vi "input.vi"(8 "error in":errorcluster, 10 "data table in":T1, 11 "UI Reference runtime in":refnum<class "UI Reference runtime.lvclass">) -> (0 "error out":errorcluster, 2 "data table out":T1, 3 "UI Reference runtime out":refnum<class "UI Reference runtime.lvclass">)   [LabVIEW 2013, in "UI Reference runtime.lvclass"]
doc: "Provides an interface for reading data from a module at runtime. While this interface performs no operations, a child should provide an override which may read from any open sessions, references, or interfaces."
uses:
  UI Reference runtime.lvclass
  <vilib>/NI/Tag Bus/table/data table.ctl
  UI Reference runtime.lvclass/UI Reference runtime.ctl
  <vilib>/NI/Tag Bus/table/data polymorphs/write many/write Doubles.vi
  <vilib>/NI/Tag Bus/table/data polymorphs/write many/write Singles.vi
  <vilib>/NI/Tag Bus/table/data polymorphs/write many/write I64s.vi
  <vilib>/NI/Tag Bus/table/data polymorphs/write many/write I32s.vi
  <vilib>/NI/Tag Bus/table/data polymorphs/write many/write I16s.vi
  <vilib>/NI/Tag Bus/table/data polymorphs/write many/write I8s.vi
  <vilib>/NI/Tag Bus/table/data polymorphs/write many/write U64s.vi
  <vilib>/NI/Tag Bus/table/data polymorphs/write many/write U32s.vi
  <vilib>/NI/Tag Bus/table/data polymorphs/write many/write U16s.vi
  <vilib>/NI/Tag Bus/table/data polymorphs/write many/write U8s.vi
  <vilib>/NI/Tag Bus/table/data polymorphs/write many/write Booleans.vi
  <vilib>/NI/Tag Bus/table/data polymorphs/write many/write Strings.vi
  <vilib>/NI/Tag Bus/table/data polymorphs/write one/write Array of Double.vi
  <vilib>/NI/Tag Bus/table/data polymorphs/write one/write Array of Single.vi
  <vilib>/NI/Tag Bus/table/data polymorphs/write one/write Array of I64.vi
  <vilib>/NI/Tag Bus/table/data polymorphs/write one/write Array of I32.vi
  <vilib>/NI/Tag Bus/table/data polymorphs/write one/write Array of I16.vi
  <vilib>/NI/Tag Bus/table/data polymorphs/write one/write Array of I8.vi
  <vilib>/NI/Tag Bus/table/data polymorphs/write one/write Array of U64.vi
  <vilib>/NI/Tag Bus/table/data polymorphs/write one/write Array of U32.vi
  <vilib>/NI/Tag Bus/table/data polymorphs/write one/write Array of U16.vi
  <vilib>/NI/Tag Bus/table/data polymorphs/write one/write Array of U8.vi
  <vilib>/NI/Tag Bus/table/data polymorphs/write one/write Array of Boolean.vi
  <vilib>/NI/Tag Bus/table/data polymorphs/write one/write Array of String.vi
  <vilib>/NI/Tag Bus/table/data table.lvlib
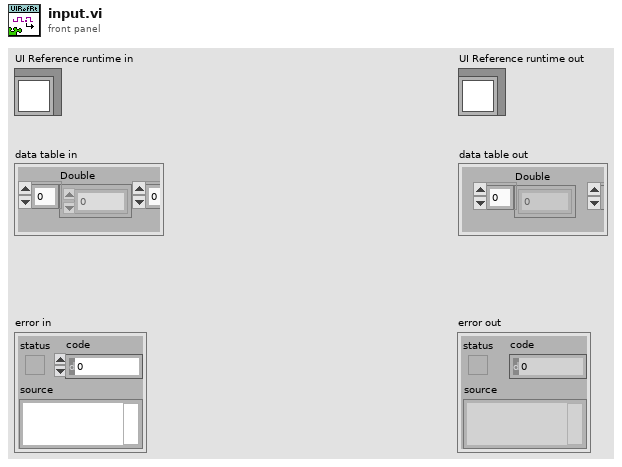
[diagram p1: front panel]
types:
  T1 = typedef "tag bus.lvlib/data table.lvlib/data table.ctl" = cluster{"Double":dbl[], "Single":sgl[], "I64":i64[], "I32":i32[], "I16":i16[], "I8":i8[], "U64":u64[], "U32":u32[], "U16":u16[], "U8":u8[], "Boolean":bool[], "String":string[], "Array of Double":cluster{"DBL Array":dbl[]}[], "Array of Single":cluster{"SGL Array":sgl[]}[], "Array of I64":cluster{"I64 Array":i64[]}[], "Array of I32":cluster{"I32 Array":i32[]}[], "Array of I16":cluster{"I16 Array":i16[]}[], "Array of I8":cluster{"I8 Array":i8[]}[], "Array of U64":cluster{"U64 Array":u64[]}[], "Array of U32":cluster{"U32 Array":u32[]}[], "Array of U16":cluster{"U16 Array":u16[]}[], "Array of U8":cluster{"U8 Array":u8[]}[], "Array of Boolean":cluster{"Boolean Array":bool[]}[], "Array of String":cluster{"String Array":string[]}[]}
  T2 = typedef "UI Reference runtime.lvclass/control index set.ctl" = cluster{"data type":T3, "control indexes":i32[], "data indexes":i32[]}
  T3 = typedef "tag bus.lvlib/tag descriptor.lvclass/Data Type.ctl" = enum16{"Double", "Single", "I64", "I32", "I16", "I8", "U64", "U32", "U16", "U8", "Boolean", "String", "Array of Double", "Array of Single", "Array of I64", "Array of I32", "Array of I16", "Array of I8", "Array of U64", "Array of U32", "Array of U16", "Array of U8", "Array of Boolean", "Array of String"}
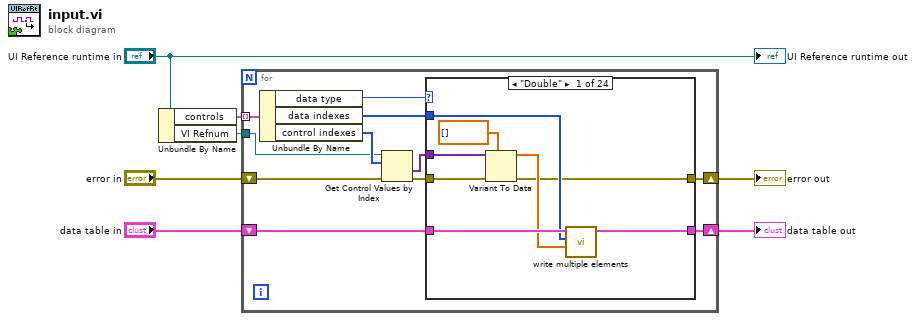
[diagram p0: block diagram]
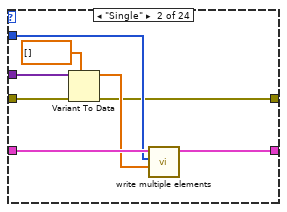
[diagram p2: hidden frame]
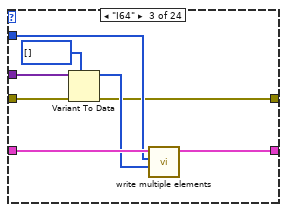
[diagram p3: hidden frame]
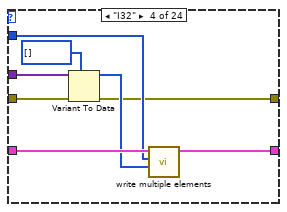
[diagram p4: hidden frame]
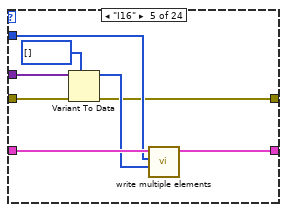
[diagram p5: hidden frame]
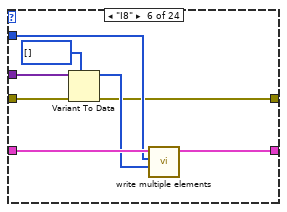
[diagram p6: hidden frame]
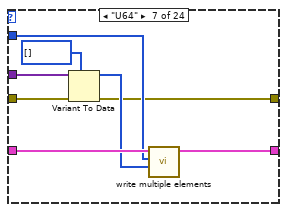
[diagram p7: hidden frame]
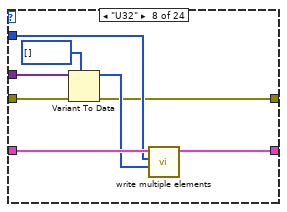
[diagram p8: hidden frame]
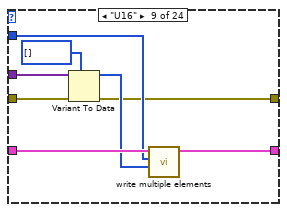
[diagram p9: hidden frame]
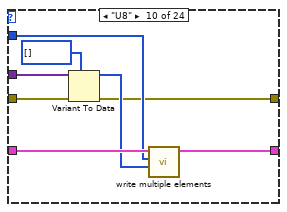
[diagram p10: hidden frame]
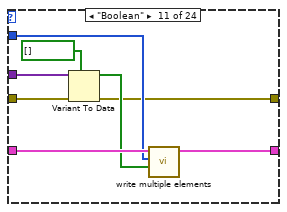
[diagram p11: hidden frame]
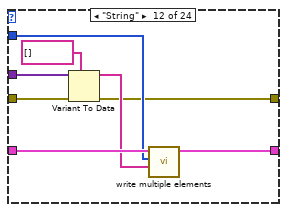
[diagram p12: hidden frame]
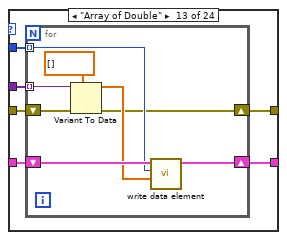
[diagram p13: hidden frame]
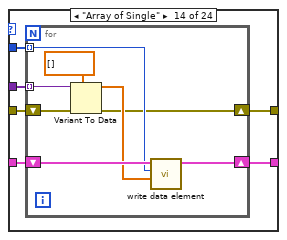
[diagram p14: hidden frame]
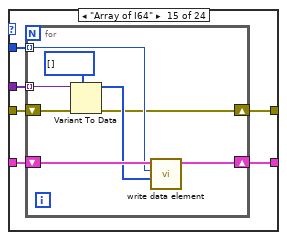
[diagram p15: hidden frame]
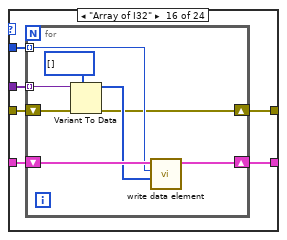
[diagram p16: hidden frame]
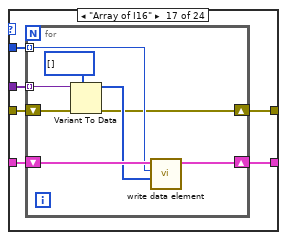
[diagram p17: hidden frame]
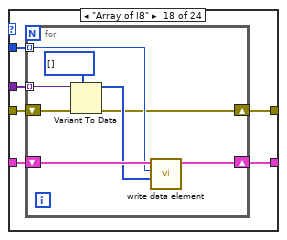
[diagram p18: hidden frame]
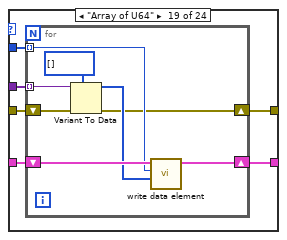
[diagram p19: hidden frame]
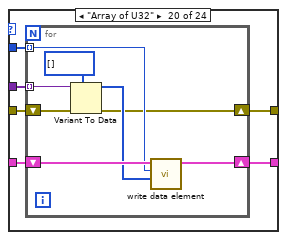
[diagram p20: hidden frame]
diagram:
  n1 = Unbundle By Name("UI Reference runtime in") -> ("controls"=w2:T2[], "VI Refnum"=w1:refnum<vi>)
  n2 = for {
    shift-right: [w10] -> w4
    shift-left: "data table in" -> [w11]
    shift-right: [w9] -> w5
    shift-left: "error in" -> [w15]
    tunnel: w2 -> [w18] mode=indexing
    tunnel: w1 -> [w8]
    n3 = Unbundle By Name(w18) -> ("data type"=w17:T3, "data indexes"=w16:i32[], "control indexes"=w14:i32[])
    n4 = Get Control Values by Index(0:w8, 1:w14, 3:w15) -> (10:w12:variant[], 11:w13:errorcluster)
    n5 = case shown="\"Double\"" w17 {
      tunnel: w16 -> [w24 w32 w40 w48 w56 w64 w72 w80 w88 w96 w104 w112 w118 w132 w146 w160 w174 w188 w202 w216 w230 w244 w258 w272]
      tunnel: w13 -> [w23 w31 w39 w47 w55 w63 w71 w79 w87 w95 w103 w111 w117 w131 w145 w159 w173 w187 w201 w215 w229 w243 w257 w271]
      tunnel: w12 -> [w22 w30 w38 w46 w54 w62 w70 w78 w86 w94 w102 w110 w116 w130 w144 w158 w172 w186 w200 w214 w228 w242 w256 w270]
      tunnel: w11 -> [w26 w34 w42 w50 w58 w66 w74 w82 w90 w98 w106 w114 w120 w134 w148 w162 w176 w190 w204 w218 w232 w246 w260 w274]
      tunnel: [w25 w33 w41 w49 w57 w65 w73 w81 w89 w97 w105 w113 w119 w133 w147 w161 w175 w189 w203 w217 w231 w245 w259 w273] -> w10
      tunnel: [w19 w27 w35 w43 w51 w59 w67 w75 w83 w91 w99 w107 w115 w129 w143 w157 w171 w185 w199 w213 w227 w241 w255 w269] -> w9
      frame "Double" {
        n6 = Variant To Data(error in=w23, type=dbl[] [], Variant=w22) -> (data=w20:dbl[], error out=w19:errorcluster)
        n7 = call-poly <vilib>:"write multiple elements.vi"("values"=w20, "indices"=w24, "data table in"=w26) -> ("data table out"=w25:T1)  [unwired: 8 in]
      }
      frame "Single" {
        n8 = Variant To Data(error in=w31, type=sgl[] [], Variant=w30) -> (data=w28:sgl[], error out=w27:errorcluster)
        n9 = call-poly <vilib>:"write multiple elements.vi"("values"=w28, "indices"=w32, "data table in"=w34) -> ("data table out"=w33:T1)  [unwired: 8 in]
      }
      frame "I64" {
        n10 = Variant To Data(error in=w39, type=i64[] [], Variant=w38) -> (data=w36:i64[], error out=w35:errorcluster)
        n11 = call-poly <vilib>:"write multiple elements.vi"("values"=w36, "indices"=w40, "data table in"=w42) -> ("data table out"=w41:T1)  [unwired: 8 in]
      }
      frame "I32" {
        n12 = Variant To Data(error in=w47, type=i32[] [], Variant=w46) -> (data=w44:i32[], error out=w43:errorcluster)
        n13 = call-poly <vilib>:"write multiple elements.vi"("values"=w44, "indices"=w48, "data table in"=w50) -> ("data table out"=w49:T1)  [unwired: 8 in]
      }
      frame "I16" {
        n14 = Variant To Data(error in=w55, type=i16[] [], Variant=w54) -> (data=w52:i16[], error out=w51:errorcluster)
        n15 = call-poly <vilib>:"write multiple elements.vi"("values"=w52, "indices"=w56, "data table in"=w58) -> ("data table out"=w57:T1)  [unwired: 8 in]
      }
      frame "I8" {
        n16 = Variant To Data(error in=w63, type=i8[] [], Variant=w62) -> (data=w60:i8[], error out=w59:errorcluster)
        n17 = call-poly <vilib>:"write multiple elements.vi"("values"=w60, "indices"=w64, "data table in"=w66) -> ("data table out"=w65:T1)  [unwired: 8 in]
      }
      frame "U64" {
        n18 = Variant To Data(error in=w71, type=u64[] [], Variant=w70) -> (data=w68:u64[], error out=w67:errorcluster)
        n19 = call-poly <vilib>:"write multiple elements.vi"("values"=w68, "indices"=w72, "data table in"=w74) -> ("data table out"=w73:T1)  [unwired: 8 in]
      }
      frame "U32" {
        n20 = Variant To Data(error in=w79, type=u32[] [], Variant=w78) -> (data=w76:u32[], error out=w75:errorcluster)
        n21 = call-poly <vilib>:"write multiple elements.vi"("values"=w76, "indices"=w80, "data table in"=w82) -> ("data table out"=w81:T1)  [unwired: 8 in]
      }
      frame "U16" {
        n22 = Variant To Data(error in=w87, type=u16[] [], Variant=w86) -> (data=w84:u16[], error out=w83:errorcluster)
        n23 = call-poly <vilib>:"write multiple elements.vi"("values"=w84, "indices"=w88, "data table in"=w90) -> ("data table out"=w89:T1)  [unwired: 8 in]
      }
      frame "U8" {
        n24 = Variant To Data(error in=w95, type=u8[] [], Variant=w94) -> (data=w92:u8[], error out=w91:errorcluster)
        n25 = call-poly <vilib>:"write multiple elements.vi"("values"=w92, "indices"=w96, "data table in"=w98) -> ("data table out"=w97:T1)  [unwired: 8 in]
      }
      frame "Boolean" {
        n26 = Variant To Data(error in=w103, type=bool[] [], Variant=w102) -> (data=w100:bool[], error out=w99:errorcluster)
        n27 = call-poly <vilib>:"write multiple elements.vi"("values"=w100, "indices"=w104, "data table in"=w106) -> ("data table out"=w105:T1)  [unwired: 8 in]
      }
      frame "String" {
        n28 = Variant To Data(error in=w111, type=string[] [], Variant=w110) -> (data=w108:string[], error out=w107:errorcluster)
        n29 = call-poly <vilib>:"write multiple elements.vi"("values"=w108, "indices"=w112, "data table in"=w114) -> ("data table out"=w113:T1)  [unwired: 8 in]
      }
      frame "Array of Double" {
        n30 = for {
          tunnel: w118 -> [w126] mode=indexing
          tunnel: w116 -> [w124] mode=indexing
          shift-right: [w121] -> w115
          shift-left: w117 -> [w125]
          shift-right: [w127] -> w119
          shift-left: w120 -> [w128]
          n31 = Variant To Data(error in=w125, type=dbl[] [], Variant=w124) -> (data=w122:dbl[], error out=w121:errorcluster)
          n32 = call-poly <vilib>:"write data element.vi"("value"=w122, "index"=w126, "data table in"=w128) -> ("data table out"=w127:T1)  [unwired: 8 in]
        }
      }
      frame "Array of Single" {
        n33 = for {
          tunnel: w132 -> [w140] mode=indexing
          tunnel: w130 -> [w138] mode=indexing
          shift-right: [w135] -> w129
          shift-left: w131 -> [w139]
          shift-right: [w141] -> w133
          shift-left: w134 -> [w142]
          n34 = Variant To Data(error in=w139, type=sgl[] [], Variant=w138) -> (data=w136:sgl[], error out=w135:errorcluster)
          n35 = call-poly <vilib>:"write data element.vi"("value"=w136, "index"=w140, "data table in"=w142) -> ("data table out"=w141:T1)  [unwired: 8 in]
        }
      }
      frame "Array of I64" {
        n36 = for {
          tunnel: w146 -> [w154] mode=indexing
          tunnel: w144 -> [w152] mode=indexing
          shift-right: [w149] -> w143
          shift-left: w145 -> [w153]
          shift-right: [w155] -> w147
          shift-left: w148 -> [w156]
          n37 = Variant To Data(error in=w153, type=i64[] [], Variant=w152) -> (data=w150:i64[], error out=w149:errorcluster)
          n38 = call-poly <vilib>:"write data element.vi"("value"=w150, "index"=w154, "data table in"=w156) -> ("data table out"=w155:T1)  [unwired: 8 in]
        }
      }
      frame "Array of I32" {
        n39 = for {
          tunnel: w160 -> [w168] mode=indexing
          tunnel: w158 -> [w166] mode=indexing
          shift-right: [w163] -> w157
          shift-left: w159 -> [w167]
          shift-right: [w169] -> w161
          shift-left: w162 -> [w170]
          n40 = Variant To Data(error in=w167, type=i32[] [], Variant=w166) -> (data=w164:i32[], error out=w163:errorcluster)
          n41 = call-poly <vilib>:"write data element.vi"("value"=w164, "index"=w168, "data table in"=w170) -> ("data table out"=w169:T1)  [unwired: 8 in]
        }
      }
      frame "Array of I16" {
        n42 = for {
          tunnel: w174 -> [w182] mode=indexing
          tunnel: w172 -> [w180] mode=indexing
          shift-right: [w177] -> w171
          shift-left: w173 -> [w181]
          shift-right: [w183] -> w175
          shift-left: w176 -> [w184]
          n43 = Variant To Data(error in=w181, type=i16[] [], Variant=w180) -> (data=w178:i16[], error out=w177:errorcluster)
          n44 = call-poly <vilib>:"write data element.vi"("value"=w178, "index"=w182, "data table in"=w184) -> ("data table out"=w183:T1)  [unwired: 8 in]
        }
      }
      frame "Array of I8" {
        n45 = for {
          tunnel: w188 -> [w196] mode=indexing
          tunnel: w186 -> [w194] mode=indexing
          shift-right: [w191] -> w185
          shift-left: w187 -> [w195]
          shift-right: [w197] -> w189
          shift-left: w190 -> [w198]
          n46 = Variant To Data(error in=w195, type=i8[] [], Variant=w194) -> (data=w192:i8[], error out=w191:errorcluster)
          n47 = call-poly <vilib>:"write data element.vi"("value"=w192, "index"=w196, "data table in"=w198) -> ("data table out"=w197:T1)  [unwired: 8 in]
        }
      }
      frame "Array of U64" {
        n48 = for {
          tunnel: w202 -> [w210] mode=indexing
          tunnel: w200 -> [w208] mode=indexing
          shift-right: [w205] -> w199
          shift-left: w201 -> [w209]
          shift-right: [w211] -> w203
          shift-left: w204 -> [w212]
          n49 = Variant To Data(error in=w209, type=u64[] [], Variant=w208) -> (data=w206:u64[], error out=w205:errorcluster)
          n50 = call-poly <vilib>:"write data element.vi"("value"=w206, "index"=w210, "data table in"=w212) -> ("data table out"=w211:T1)  [unwired: 8 in]
        }
      }
      frame "Array of U32" {
        n51 = for {
          tunnel: w216 -> [w224] mode=indexing
          tunnel: w214 -> [w222] mode=indexing
          shift-right: [w219] -> w213
          shift-left: w215 -> [w223]
          shift-right: [w225] -> w217
          shift-left: w218 -> [w226]
          n52 = Variant To Data(error in=w223, type=u32[] [], Variant=w222) -> (data=w220:u32[], error out=w219:errorcluster)
          n53 = call-poly <vilib>:"write data element.vi"("value"=w220, "index"=w224, "data table in"=w226) -> ("data table out"=w225:T1)  [unwired: 8 in]
        }
      }
      frame "Array of U16" {
        n54 = for {
          tunnel: w230 -> [w238] mode=indexing
          tunnel: w228 -> [w236] mode=indexing
          shift-right: [w233] -> w227
          shift-left: w229 -> [w237]
          shift-right: [w239] -> w231
          shift-left: w232 -> [w240]
          n55 = Variant To Data(error in=w237, type=u16[] [], Variant=w236) -> (data=w234:u16[], error out=w233:errorcluster)
          n56 = call-poly <vilib>:"write data element.vi"("value"=w234, "index"=w238, "data table in"=w240) -> ("data table out"=w239:T1)  [unwired: 8 in]
        }
      }
      frame "Array of U8" {
        n57 = for {
          tunnel: w244 -> [w252] mode=indexing
          tunnel: w242 -> [w250] mode=indexing
          shift-right: [w247] -> w241
          shift-left: w243 -> [w251]
          shift-right: [w253] -> w245
          shift-left: w246 -> [w254]
          n58 = Variant To Data(error in=w251, type=u8[] [], Variant=w250) -> (data=w248:u8[], error out=w247:errorcluster)
          n59 = call-poly <vilib>:"write data element.vi"("value"=w248, "index"=w252, "data table in"=w254) -> ("data table out"=w253:T1)  [unwired: 8 in]
        }
      }
      frame "Array of Boolean" {
        n60 = for {
          tunnel: w258 -> [w261] mode=indexing
          tunnel: w256 -> [w265] mode=indexing
          shift-right: [w262] -> w255
          shift-left: w257 -> [w266]
          shift-right: [w267] -> w259
          shift-left: w260 -> [w268]
          n61 = Variant To Data(error in=w266, type=bool[] [], Variant=w265) -> (data=w263:bool[], error out=w262:errorcluster)
          n62 = call-poly <vilib>:"write data element.vi"("value"=w263, "index"=w261, "data table in"=w268) -> ("data table out"=w267:T1)  [unwired: 8 in]
        }
      }
      frame "Array of String" {
        n63 = for {
          tunnel: w272 -> [w275] mode=indexing
          tunnel: w270 -> [w279] mode=indexing
          shift-right: [w276] -> w269
          shift-left: w271 -> [w280]
          shift-right: [w281] -> w273
          shift-left: w274 -> [w282]
          n64 = Variant To Data(error in=w280, type=string[] [], Variant=w279) -> (data=w277:string[], error out=w276:errorcluster)
          n65 = call-poly <vilib>:"write data element.vi"("value"=w277, "index"=w275, "data table in"=w282) -> ("data table out"=w281:T1)  [unwired: 8 in]
        }
      }
    }
  }
  "error out" <- w5
  "data table out" <- w4
  "UI Reference runtime out" <- "UI Reference runtime in"
